vi "Scan Setup.vi"(8 "error in (no error)":errorcluster, 11 "Wavelength Digikröm in":refnum<class "Wavelength Digikröm.lvclass">) -> (0 "error out":errorcluster, 3 "Wavelength Digikröm out":refnum<class "Wavelength Digikröm.lvclass">)   [LabVIEW 2017, in "Wavelength Digikröm.lvclass"]
doc: "Configure the instrument based on the class member data. This step comes after the user has closed the \"Scan Setup\" window and before the actual scan -- so instruments are configured with the user's specified settings."
uses:
  Scanner/Scanner.lvclass
  Global/GPIB Numbers.vi
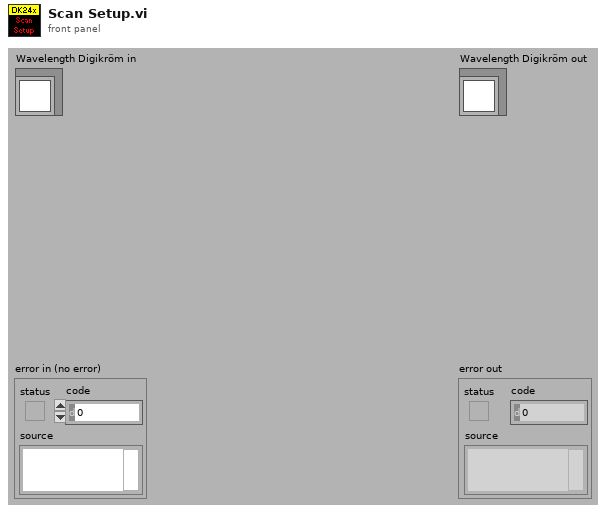
[diagram p1: front panel]
types:
  T1 = typedef "GPIB Type Def.ctl" = cluster{"Name":string, "bus":dbl, "GPIB":dbl, "GPIB as string":string, "byte":i32, "VISA Resource Name":refnum<visa-resource-name>}
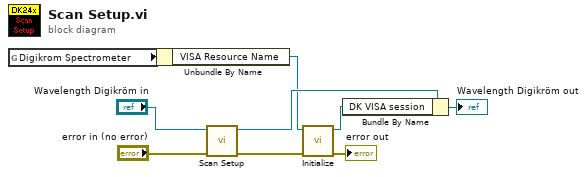
[diagram p0: block diagram]
diagram:
  n1 = global read "GPIB Numbers.vi" "Digikrom Spectrometer"() -> (w2:T1)
  n2 = Unbundle By Name(w2) -> ("VISA Resource Name"=w1:refnum<visa-resource-name>)
  n3 = call-parent "Scan Setup.vi"("error in (no error)"="error in (no error)", "Scanner in"="Wavelength Digikröm in") -> ("error out"=w4:errorcluster, "Scanner out"=w9:refnum<class "Wavelength Digikröm.lvclass">)  [unwired: 8 out]
  n4 = call "Initialize.vi"("error in (no error)"=w4, "VISA resource name"=w1) -> ("error out"=→"error out":errorcluster, "VISA resource name out"=w5:refnum<visa-resource-name>)  [unwired: 8 out]
  n5 = Bundle By Name(cluster=w9, "DK VISA session"=w5) -> (→"Wavelength Digikröm out":refnum<class "Wavelength Digikröm.lvclass">)
